vi "ep_Speed Estimation for Single Motor.vi"(0 "signals":dbl[][](array[numeric]), 2 "reset? (F)":bool, 5 "fundamental frequency [Hz]":dbl format="%#_13g", 7 "nominal frequency":enum16{"50 Hz", "60 Hz"}(ring), 9 "nameplate speed":T1, 11 "error in (no error)":errorcluster, 12 "initial conditions":T2={"SVAF state"={"space vector amplitude"=0.0, "hilbert state"={"delay conditions"=[], "filter conditions"=[]}}, "zoom FFT state"={"phase state"=0.0, "zoom FFT state"={"zoom settings state"={"zoom"=0, "stop band attenuation"=enum."84 dB", "alias protect in final transition"=FALSE, "oversampling ratio"=0.0}, "SML Decimation Filter (complex input) state"={"decimation settings state"={"M"=0, "stop band attenuation"=enum."84 dB", "alias protect in transition band"=FALSE, "oversampling ratio"=0.0}, "counter for garbage samples state"=0, "sml_Parameter Setting for Zoom Factor state"={"filter length * interpolation state"=0, "interpolation state"=0, "comb filter order state"=0, "CFIR par state"={"h"=[], "M"=0, "N"=0}, "LFIR par state"={"h"=[], "M"=0, "N"=0}, "CIC Stages state"=0}, "aal_CIC (complex input) state"={"aal_cascaded moving average (complex input) state"={"states"=[], "circular buffers state"=[], "circular buffer counter state"=0}, "aal_moving average with decimation by order (complex input) state"={"residue result state"=0.0+0.0i, "processed data counter state"=0}}, "sml_Cascaded Decimation Filter (complex input) CFIR state"={"unprocessed data state"=[], "final conditions state"=[], "sml_M-1 Decimator with IC (complex input) state"={"coefficients in reverse order state"=[], "max index for coefficients state"=0}}, "sml_Cascaded Decimation Filter (complex input) LFIR state"={"unprocessed data state"=[], "final conditions state"=[], "sml_M-1 Decimator with IC (complex input) state"={"coefficients in reverse order state"=[], "max index for coefficients state"=0}}}, "ma_SML Data Packing (complex input) state"={"array getting packed state"=[], "last array processed state"=[], "index state"=0, "packing parameters state"={0, "size"=0}}}, "FFT{X} [Vrms]"=[]}, "speed state"={"speed [RPM]"=nan, "slip"=nan}, "speed estimation settings"={"% overlap"=0.0, "algorithm"=enum."3-phase signals"}, "filter information"={"coefficients"=[], "order"=0}, "zoom FFT settings"={"FFT settings"={"window"=0, "Window Size"=0, "FFT Size"=0, "%overlap"=0.0}, "zoom settings"={"zoom"=0, "stop band attenuation"=enum."84 dB", "alias protect in final transition"=FALSE, "oversampling ratio"=0.0}, "other settings"={"fmod"=0.0, "f0"=0.0, "df"=0.0, "oidx"=0, "olen"=0}, "iterations"=0, "max block size"=0, "fs"=0.0}, "last valid window"=0, "fund. frequency for averager"=[]} {"zoom FFT settings"."FFT settings"."window" items=["Rectangle"=0, "Hanning"=1, "Hamming"=2, "Blackman-Harris"=3, "Exact Blackman"=4, "Blackman"=5, "Flat Top"=6, "4 Term B-Harris "=7, "7 Term B-Harris"=8, "Low Sidelobe"=9, "Blackman Nuttall"=11, "Triangle"=30, "Bartlett-Hanning"=31, "Bohman"=32, "Parzen"=33, "Welch"=34, "Kaiser"=60, "Dolph-Chebyshev"=61, "Gaussian"=62]}) -> (3 "new speed available?":bool, 4 "speed [RPM]":dbl, 6 "slip":dbl, 14 "final conditions":T2={"SVAF state"={"space vector amplitude"=0.0, "hilbert state"={"delay conditions"=[], "filter conditions"=[]}}, "zoom FFT state"={"phase state"=0.0, "zoom FFT state"={"zoom settings state"={"zoom"=0, "stop band attenuation"=enum."84 dB", "alias protect in final transition"=FALSE, "oversampling ratio"=0.0}, "SML Decimation Filter (complex input) state"={"decimation settings state"={"M"=0, "stop band attenuation"=enum."84 dB", "alias protect in transition band"=FALSE, "oversampling ratio"=0.0}, "counter for garbage samples state"=0, "sml_Parameter Setting for Zoom Factor state"={"filter length * interpolation state"=0, "interpolation state"=0, "comb filter order state"=0, "CFIR par state"={"h"=[], "M"=0, "N"=0}, "LFIR par state"={"h"=[], "M"=0, "N"=0}, "CIC Stages state"=0}, "aal_CIC (complex input) state"={"aal_cascaded moving average (complex input) state"={"states"=[], "circular buffers state"=[], "circular buffer counter state"=0}, "aal_moving average with decimation by order (complex input) state"={"residue result state"=0.0+0.0i, "processed data counter state"=0}}, "sml_Cascaded Decimation Filter (complex input) CFIR state"={"unprocessed data state"=[], "final conditions state"=[], "sml_M-1 Decimator with IC (complex input) state"={"coefficients in reverse order state"=[], "max index for coefficients state"=0}}, "sml_Cascaded Decimation Filter (complex input) LFIR state"={"unprocessed data state"=[], "final conditions state"=[], "sml_M-1 Decimator with IC (complex input) state"={"coefficients in reverse order state"=[], "max index for coefficients state"=0}}}, "ma_SML Data Packing (complex input) state"={"array getting packed state"=[], "last array processed state"=[], "index state"=0, "packing parameters state"={0, "size"=0}}}, "FFT{X} [Vrms]"=[]}, "speed state"={"speed [RPM]"=nan, "slip"=nan}, "speed estimation settings"={"% overlap"=0.0, "algorithm"=enum."3-phase signals"}, "filter information"={"coefficients"=[], "order"=0}, "zoom FFT settings"={"FFT settings"={"window"=0, "Window Size"=0, "FFT Size"=0, "%overlap"=0.0}, "zoom settings"={"zoom"=0, "stop band attenuation"=enum."84 dB", "alias protect in final transition"=FALSE, "oversampling ratio"=0.0}, "other settings"={"fmod"=0.0, "f0"=0.0, "df"=0.0, "oidx"=0, "olen"=0}, "iterations"=0, "max block size"=0, "fs"=0.0}, "last valid window"=0, "fund. frequency for averager"=[]} {"zoom FFT settings"."FFT settings"."window" items=["Rectangle"=0, "Hanning"=1, "Hamming"=2, "Blackman-Harris"=3, "Exact Blackman"=4, "Blackman"=5, "Flat Top"=6, "4 Term B-Harris "=7, "7 Term B-Harris"=8, "Low Sidelobe"=9, "Blackman Nuttall"=11, "Triangle"=30, "Bartlett-Hanning"=31, "Bohman"=32, "Parzen"=33, "Welch"=34, "Kaiser"=60, "Dolph-Chebyshev"=61, "Gaussian"=62]}, 15 "error out":errorcluster)   [LabVIEW 2014, in "NI_EP_Motor Monitoring.lvlib"]
uses:
  <vilib>/addons/Electrical Power/Motor Monitoring/NI_EP_Motor Monitoring.lvlib
  <vilib>/addons/Electrical Power/Motor Monitoring/subVIs/ep_Initial Conditions for Speed Estimation.ctl
  <vilib>/addons/Electrical Power/Motor Monitoring/subVIs/ep_Demodulation Algorithm.ctl
  <vilib>/addons/Electrical Power/Motor Monitoring/subVIs/ep_Zoom FFT Settings.ctl
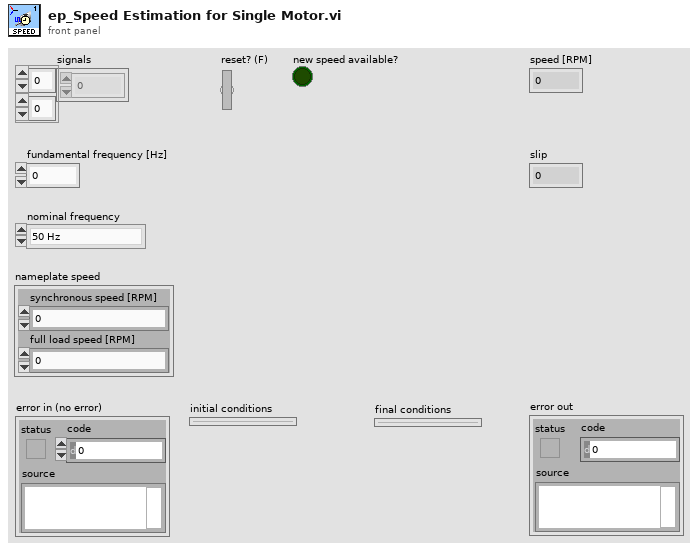
[diagram p1: front panel]
types:
  T1 = cluster{"synchronous speed [RPM]":dbl, "full load speed [RPM]":dbl}
  T2 = typedef "NI_EP_Motor Monitoring.lvlib/ep_Initial Conditions for Speed Estimation.ctl" = cluster{"SVAF state":cluster{"space vector amplitude":dbl, "hilbert state":cluster{"delay conditions":dbl[], "filter conditions":dbl[]}}, "zoom FFT state":cluster{"phase state":dbl, "zoom FFT state":cluster{"zoom settings state":cluster{"zoom":i32, "stop band attenuation":enum16{"84 dB", "96 dB", "120 dB"}, "alias protect in final transition":bool, "oversampling ratio":dbl}, "SML Decimation Filter (complex input) state":cluster{"decimation settings state":cluster{"M":i32, "stop band attenuation":enum16{"84 dB", "96 dB", "120 dB"}, "alias protect in transition band":bool, "oversampling ratio":dbl}, "counter for garbage samples state":i32, "sml_Parameter Setting for Zoom Factor state":cluster{"filter length * interpolation state":i32, "interpolation state":i32, "comb filter order state":i32, "CFIR par state":cluster{"h":dbl[], "M":i32, "N":i32}, "LFIR par state":cluster{"h":dbl[], "M":i32, "N":i32}, "CIC Stages state":i32}, "aal_CIC (complex input) state":cluster{"aal_cascaded moving average (complex input) state":cluster{"states":cdb[], "circular buffers state":cdb[][], "circular buffer counter state":i32}, "aal_moving average with decimation by order (complex input) state":cluster{"residue result state":cdb, "processed data counter state":i32}}, "sml_Cascaded Decimation Filter (complex input) CFIR state":cluster{"unprocessed data state":cdb[], "final conditions state":cdb[][], "sml_M-1 Decimator with IC (complex input) state":cluster{"coefficients in reverse order state":dbl[], "max index for coefficients state":i32}}, "sml_Cascaded Decimation Filter (complex input) LFIR state":cluster{"unprocessed data state":cdb[], "final conditions state":cdb[][], "sml_M-1 Decimator with IC (complex input) state":cluster{"coefficients in reverse order state":dbl[], "max index for coefficients state":i32}}}, "ma_SML Data Packing (complex input) state":cluster{"array getting packed state":cdb[], "last array processed state":cdb[], "index state":i32, "packing parameters state":cluster{i32, "size":i32}}}, "FFT{X} [Vrms]":cdb[]}, "speed state":cluster{"speed [RPM]":dbl, "slip":dbl}, "speed estimation settings":cluster{"% overlap":dbl, "algorithm":T3}, "filter information":cluster{"coefficients":dbl[], "order":i32}, "zoom FFT settings":T4, "last valid window":i32, "fund. frequency for averager":dbl[]}
  T3 = typedef "NI_EP_Motor Monitoring.lvlib/ep_Demodulation Algorithm.ctl" = enum16{"1-phase signal", "3-phase signals"}
  T4 = typedef "NI_EP_Motor Monitoring.lvlib/ep_Zoom FFT Settings.ctl" = cluster{"FFT settings":cluster{"window":u16, "Window Size":i32, "FFT Size":i32, "%overlap":dbl}, "zoom settings":cluster{"zoom":i32, "stop band attenuation":enum16{"84 dB", "96 dB", "120 dB"}, "alias protect in final transition":bool, "oversampling ratio":dbl}, "other settings":cluster{"fmod":dbl, "f0":dbl, "df":dbl, "oidx":i32, "olen":i32}, "iterations":i32, "max block size":i32, "fs":dbl}
  T5 = cluster{"space vector amplitude":dbl, "hilbert state":cluster{"delay conditions":dbl[], "filter conditions":dbl[]}}
  T6 = cluster{"phase state":dbl, "zoom FFT state":cluster{"zoom settings state":cluster{"zoom":i32, "stop band attenuation":enum16{"84 dB", "96 dB", "120 dB"}, "alias protect in final transition":bool, "oversampling ratio":dbl}, "SML Decimation Filter (complex input) state":cluster{"decimation settings state":cluster{"M":i32, "stop band attenuation":enum16{"84 dB", "96 dB", "120 dB"}, "alias protect in transition band":bool, "oversampling ratio":dbl}, "counter for garbage samples state":i32, "sml_Parameter Setting for Zoom Factor state":cluster{"filter length * interpolation state":i32, "interpolation state":i32, "comb filter order state":i32, "CFIR par state":cluster{"h":dbl[], "M":i32, "N":i32}, "LFIR par state":cluster{"h":dbl[], "M":i32, "N":i32}, "CIC Stages state":i32}, "aal_CIC (complex input) state":cluster{"aal_cascaded moving average (complex input) state":cluster{"states":cdb[], "circular buffers state":cdb[][], "circular buffer counter state":i32}, "aal_moving average with decimation by order (complex input) state":cluster{"residue result state":cdb, "processed data counter state":i32}}, "sml_Cascaded Decimation Filter (complex input) CFIR state":cluster{"unprocessed data state":cdb[], "final conditions state":cdb[][], "sml_M-1 Decimator with IC (complex input) state":cluster{"coefficients in reverse order state":dbl[], "max index for coefficients state":i32}}, "sml_Cascaded Decimation Filter (complex input) LFIR state":cluster{"unprocessed data state":cdb[], "final conditions state":cdb[][], "sml_M-1 Decimator with IC (complex input) state":cluster{"coefficients in reverse order state":dbl[], "max index for coefficients state":i32}}}, "ma_SML Data Packing (complex input) state":cluster{"array getting packed state":cdb[], "last array processed state":cdb[], "index state":i32, "packing parameters state":cluster{i32, "size":i32}}}, "FFT{X} [Vrms]":cdb[]}
  T7 = cluster{"maximum frequency [Hz]":dbl, "slip error allowance":dbl, "minimum points for peak search":dbl, "accuracy of fs":dbl, "difference?":bool, " fs harmonics order":i32, "fs forbidden range":dbl, "p3:p1 valid significance ratio":dbl, "ratio for significance weighting":dbl, "significance weighting":dbl}
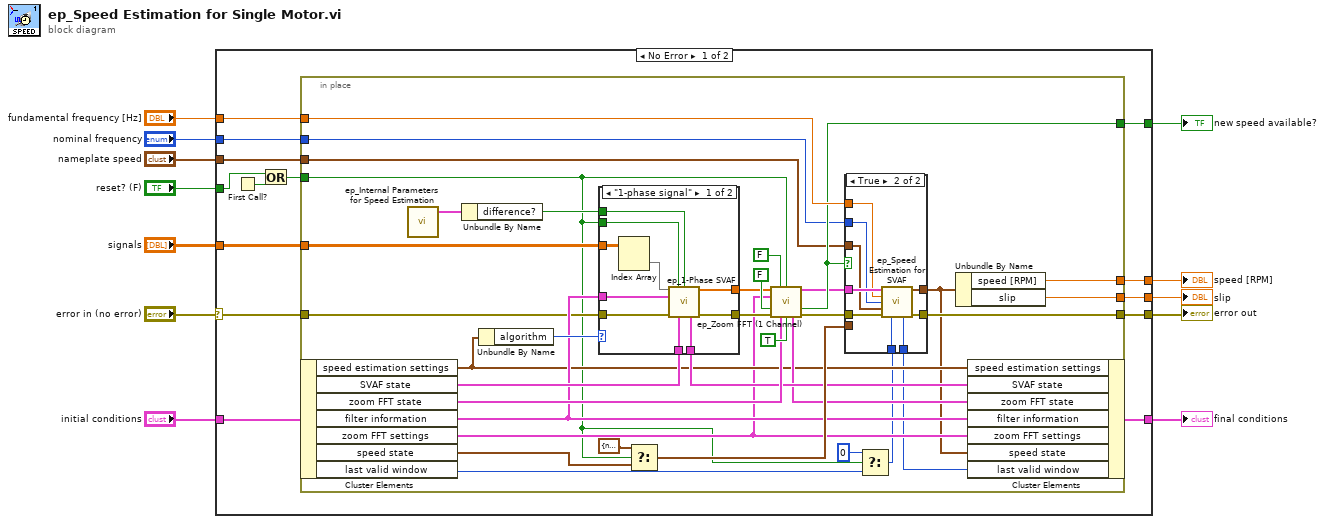
[diagram p0: block diagram]
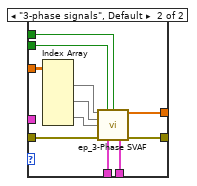
[diagram p3: hidden frame]
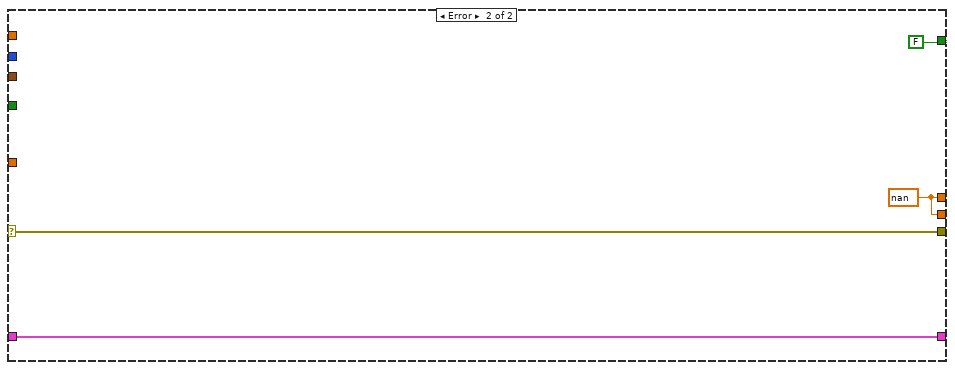
[diagram p4: hidden frame]
diagram:
  n1 = case shown="No Error" "error in (no error)" {
    selector: "error in (no error)" -> [w23 w98]
    tunnel: [w19 w98] -> w11
    tunnel: "reset? (F)" -> [w25 _]
    tunnel: "signals" -> [w24 _]
    tunnel: [w18 FALSE] -> w8
    tunnel: "nameplate speed" -> [w21 _]
    tunnel: "initial conditions" -> [w17 w96]
    tunnel: [w16 w96] -> w5
    tunnel: "fundamental frequency [Hz]" -> [w20 _]
    tunnel: "nominal frequency" -> [w15 _]
    tunnel: [w14 w95] -> w2
    tunnel: [w13 w95] -> w1
    frame No Error {
      n2 = First Call?() -> (First Call?: T/F=w26:bool)
      n3 = Or(x=w25, y=w26) -> (x .or. y?=w22:bool)
      n4 = in-place {
        in-place-border: w24 -> [w59]
        in-place-border: w23 -> [w31]
        in-place-border: w22 -> [w27]
        in-place-border: w21 -> [w39]
        in-place-border: w20 -> [w54]
        in-place-border: [w52] -> w19
        in-place-border: [w51] -> w18
        in-place-border: w15 -> [w40]
        in-place-border: [w35] -> w14
        in-place-border: [w34] -> w13
        n5 = in-place-cluster #1(w17) -> ("speed estimation settings"=w42:cluster{"% overlap":dbl, "algorithm":T3}, "SVAF state"=w49:T5, "zoom FFT state"=w48:T6, "filter information"=w43:cluster{"coefficients":dbl[], "order":i32}, "zoom FFT settings"=w41:T4, "speed state"=w45:cluster{"speed [RPM]":dbl, "slip":dbl}, "last valid window"=w30:i32)
        n6 = call <vilib>:"ep_Internal Parameters for Speed Estimation.vi"() -> ("internal parameters for speed estimation"=w38:T7)  [unwired: 11 in]
        n7 = Unbundle By Name(w38) -> ("difference?"=w37:bool)
        n8 = Unbundle By Name(w42) -> ("algorithm"=w44:T3)
        n9 = case shown="\"1-phase signal\"" w44 {
          tunnel: w59 -> [w83 w94]
          tunnel: w27 -> [w80 w85]
          tunnel: w49 -> [w79 w90]
          tunnel: [w78 w89] -> w47
          tunnel: [w74 w88] -> w58
          tunnel: w31 -> [w76 w87]
          tunnel: [w77 w86] -> w57
          tunnel: w37 -> [w81 w84]
          tunnel: w43 -> [w75 _]
          frame "1-phase signal" {
            n10 = Index Array(array=w83) -> (element=w82:dbl[])  [unwired: 2 in]
            n11 = call <vilib>:"ep_1-Phase SVAF.vi"("signal"=w82, "reset? (F)"=w80, "difference? (T)"=w81, "filter information"=w75, "error in (no error)"=w76, "previous SVAF state"=w79) -> ("SVAF signal"=w74:dbl[], "next SVAF state"=w78:T5, "error out"=w77:errorcluster)  [unwired: 7 in]
          }
          frame "3-phase signals", Default {
            n12 = Index Array(array=w94) -> (element #1=w93:dbl[], element #2=w92:dbl[], element #3=w91:dbl[])  [unwired: 6 in]
            n13 = call <vilib>:"ep_3-Phase SVAF.vi"("phase A"=w93, "reset? (F)"=w85, "difference? (T)"=w84, "phase B"=w92, "phase C"=w91, "error in (no error)"=w87, "previous SVAF state"=w90) -> ("SVAF signal"=w88:dbl[], "next SVAF state"=w89:T5, "error out"=w86:errorcluster)  [unwired: 6 in]
          }
        }
        n14 = Select(t=cluster{"speed [RPM]":dbl, "slip":dbl} {"speed [RPM]"=nan, "slip"=nan}, s=w27, f=w45) -> (s? t:f=w55:cluster{"speed [RPM]":dbl, "slip":dbl})
        n15 = call <vilib>:"ep_Zoom FFT (1 Channel).vi"("signal"=w58, "phase output? (F)"=FALSE, "reset? (F)"=w27, "zoom FFT settings"=w41, "dB on? (T)"=FALSE, "error in (no error)"=w57, "zoom FFT state in"=w48, "demodulated? (F)"=TRUE) -> ("FFT magnitude"=w32:cluster{"f0":dbl, "df":dbl, "magnitude":dbl[]}, "spectrum ready?"=w51:bool, "zoom FFT state out"=w46:T6, "error out"=w53:errorcluster)  [unwired: 3 in, 1 out]
        n16 = Select(t=0, s=w27, f=w30) -> (s? t:f=w29:i32)
        n17 = case shown="True" w51 {
          tunnel: w55 -> [w64 _]
          tunnel: [w64 w68] -> w36
          tunnel: w32 -> [_ w73]
          tunnel: w39 -> [_ w67]
          tunnel: w54 -> [_ w72]
          tunnel: w53 -> [w63 w70]
          tunnel: [w63 w69] -> w52
          tunnel: w40 -> [_ w71]
          tunnel: w29 -> [w62 w66]
          tunnel: [w62 w65] -> w33
          frame False {
          }
          frame True {
            n18 = call <vilib>:"ep_Speed Estimation for SVAF.vi"("SVAF spectrum"=w73, "fundamental frequency [Hz]"=w72, "nominal frequency"=w71, "nameplate speed"=w67, "error in (no error)"=w70, "last valid window"=w66) -> ("speed data"=w68:cluster{"speed [RPM]":dbl, "slip":dbl}, "current valid window"=w65:i32, "error out"=w69:errorcluster)  [unwired: 7 in]
          }
        }
        n19 = Unbundle By Name(w36) -> ("speed [RPM]"=w35:dbl, "slip"=w34:dbl)
        n20 = in-place-cluster #1("speed estimation settings"=w42, "SVAF state"=w47, "zoom FFT state"=w46, "filter information"=w43, "zoom FFT settings"=w41, "speed state"=w36, "last valid window"=w33) -> (w16:T2)
      }
    }
    frame Error {
      w95 = nan ("speed [RPM]")
    }
  }
  "error out" <- w11
  "new speed available?" <- w8
  "final conditions" <- w5
  "speed [RPM]" <- w2
  "slip" <- w1
